vi "Publish Drive PID.vi"(11 "Drive with PID":T1={"Max Speed"=0.7, "P/I/D"=[1.0, 0.0, 0.01], "Min Speed"=0.4, "Accel Distance"=64.0}) -> ()   [LabVIEW 2017]
uses:
  <vilib>/Rock Robotics/Network Tables/NT Write Number.vi
  <vilib>/Rock Robotics/Network Tables/NT Write Numeric Array.vi
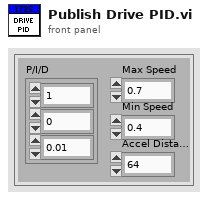
[diagram p1: front panel]
types:
  T1 = cluster{"Max Speed":dbl, "P/I/D":dbl[], "Min Speed":dbl, "Accel Distance":dbl}
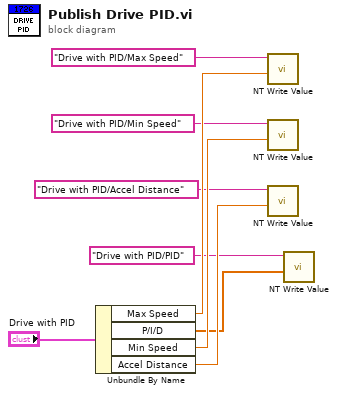
[diagram p0: block diagram]
diagram:
  n1 = Unbundle By Name("Drive with PID") -> ("Max Speed"=w7:dbl, "P/I/D"=w6:dbl[], "Min Speed"=w9:dbl, "Accel Distance"=w8:dbl)
  n2 = call-poly <vilib>:"NT Write Value.vi"("Numeric"=w7, "Name"="Drive with PID/Max Speed") -> ()  [unwired: 9 in, 1 out]
  n3 = call-poly <vilib>:"NT Write Value.vi"("Numeric"=w9, "Name"="Drive with PID/Min Speed") -> ()  [unwired: 9 in, 1 out]
  n4 = call-poly <vilib>:"NT Write Value.vi"("Numeric"=w8, "Name"="Drive with PID/Accel Distance") -> ()  [unwired: 9 in, 1 out]
  n5 = call-poly <vilib>:"NT Write Value.vi"("Numeric Array"=w6, "Name"="Drive with PID/PID") -> ()  [unwired: 9 in, 1 out]
